vi "Draw Triangle.vi"(6 "Colour":u32(colorbox), 8 "Point 3":T1, 9 "Point 2":T1, 10 "Point 1":T1, 11 "Pixel Data in":u32[][](array[numeric])) -> (3 "Pixel Data out":u32[][](array[numeric]))   [LabVIEW 2020, in "Raster.lvlib"]
uses:
  Raster.lvlib
  Point 2D.ctl
  Utility/Delta Time.vi
  <vilib>/Utility/High Resolution Relative Seconds.vi
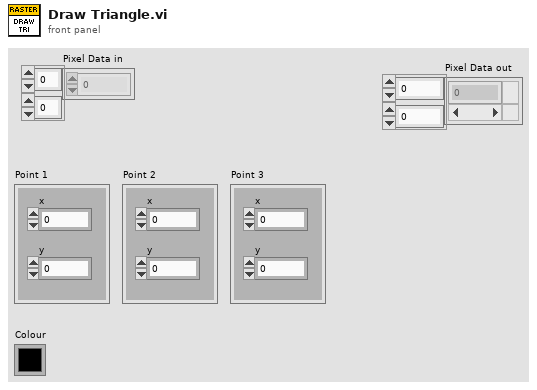
[diagram p1: front panel]
types:
  T1 = typedef "Raster.lvlib/Point 2D.ctl" = cluster{"x":i32, "y":i32}
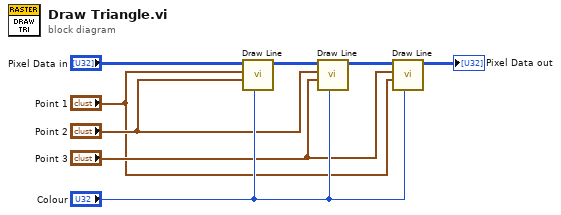
[diagram p0: block diagram]
diagram:
  n1 = call "Draw Line.vi"("Colour"="Colour", "Point 2"="Point 2", "Point 1"="Point 1", "Pixel Data in"="Pixel Data in") -> ("Pixel Data out"=w8:u32[][])  [unwired: 7 in]
  n2 = call "Draw Line.vi"("Colour"="Colour", "Point 2"="Point 3", "Point 1"="Point 2", "Pixel Data in"=w8) -> ("Pixel Data out"=w7:u32[][])  [unwired: 7 in]
  n3 = call "Draw Line.vi"("Colour"="Colour", "Point 2"="Point 1", "Point 1"="Point 3", "Pixel Data in"=w7) -> ("Pixel Data out"=→"Pixel Data out":u32[][])  [unwired: 7 in]
